vi "Generate AC Measurement Waveform.vi"(6 "hardware commands sync queue":T1, 7 "Voltage(volts)":dbl, 8 "error in":errorcluster, 9 "Frequency":dbl, 10 "DAQmx product name":string, 11 "DSG task in":refnum<k21>) -> (0 "error out":errorcluster, 3 "DSG task out":refnum<k21>)   [LabVIEW 2021]
uses:
  controls/Sync Commands Queue Ref.ctl
  controls/Sync Commands.ctl
  <vilib>/addons/_NISVFA/_Generation/Signal Generation/SV Signal/sv_System Timing Model.ctl
  <vilib>/DAQmx/write.llb/DAQmx Write (Analog 1D Wfm NChan NSamp).vi
  <vilib>/addons/_NISVFA/_Generation/Signal Generation/SV Sinusoid/SV Sinusoid.lvclass
  C:/Program Files/National Instruments/LabVIEW 2021/vi.lib/addons/_NISVFA/_Generation/Signal Generation/SV Signal/SV Signal.lvclass
  <vilib>/addons/_NISVFA/_Generation/Signal Generation/SV Sinusoid/Configure Sine.vi
  <vilib>/addons/_NISVFA/_Generation/Signal Generation/SV Signal/Write Sample Rate.vi
  <vilib>/addons/_NISVFA/_Generation/Signal Generation/SV Signal/Write System Timing Model.vi
  <vilib>/addons/_NISVFA/_Generation/Signal Generation/SV Signal/Write Ramp Parameters.vi
  <vilib>/DAQmx/miscellaneous.llb/DAQmx Fill In Error Info.vi
  <resource>/objmgr/daqmx.rc
  <vilib>/addons/_NISVFA/_Generation/Signal Generation/SV Signal/SV Signal.lvclass
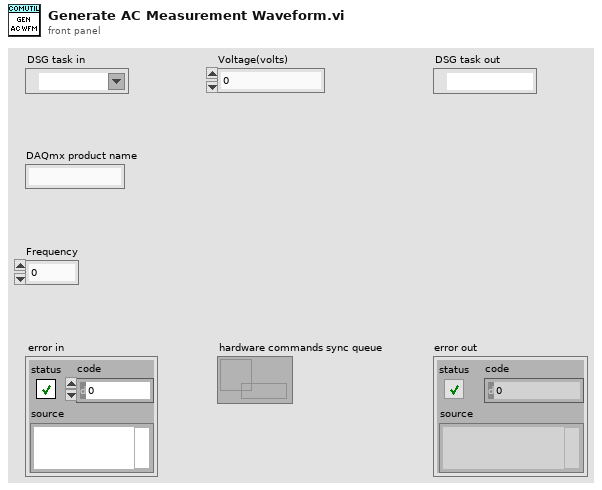
[diagram p1: front panel]
types:
  T1 = typedef "Sync Commands Queue Ref.ctl" = refnum<queue>
  T2 = typedef "Sync Commands.ctl" = enum16{"NoAction", "GenerationStarted", "AcquisitionCompleted", "GenerationErrored"}
  T3 = cluster{"profile":enum16{"Linear", "Half cosine"}, "durations [s]":cluster{"ramp-up":dbl, "transition":dbl, "ramp-down":dbl}}
  T4 = typedef "SV Signal.lvclass/sv_System Timing Model.ctl" = i64
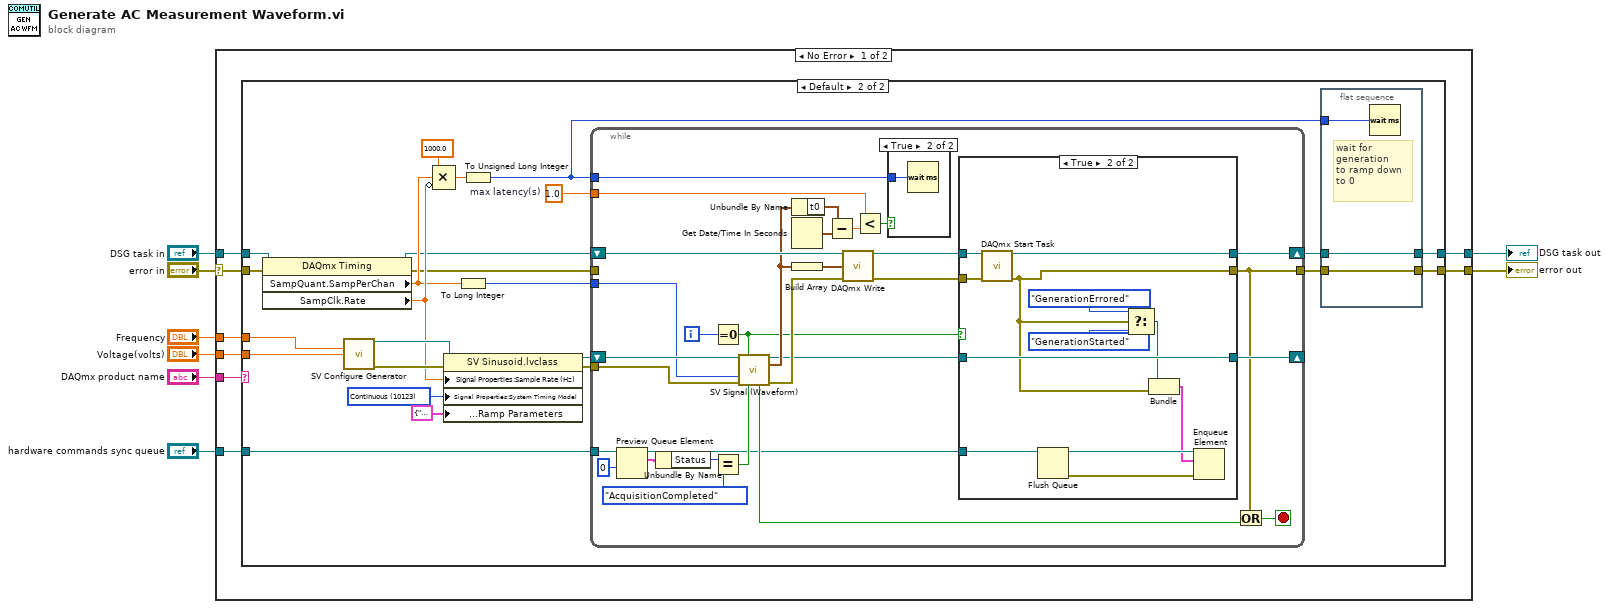
[diagram p0: block diagram]
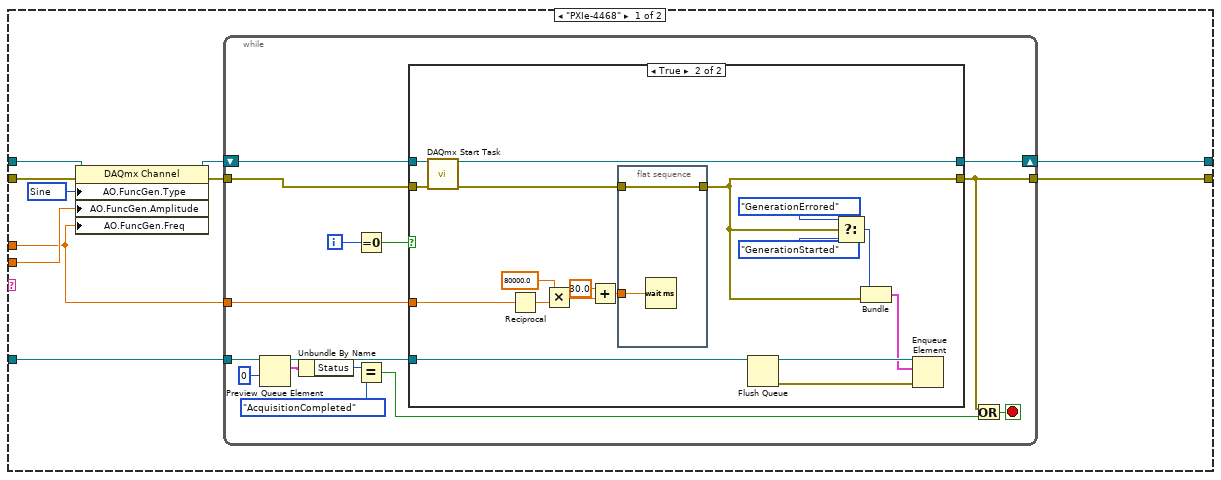
[diagram p2: hidden frame]
diagram:
  n1 = case shown="No Error" "error in" {
    selector: "error in" -> [w16 w138]
    tunnel: [w15 w137] -> w7
    tunnel: [w14 w138] -> w6
    tunnel: "DSG task in" -> [w11 w137]
    tunnel: "hardware commands sync queue" -> [w13 _]
    tunnel: "DAQmx product name" -> [w10 _]
    tunnel: "Frequency" -> [w9 _]
    tunnel: "Voltage(volts)" -> [w12 _]
    frame No Error {
      n2 = case shown="Default" w10 {
        tunnel: w16 -> [w20 w87]
        tunnel: w11 -> [w22 w83]
        tunnel: [w25 w71] -> w15
        tunnel: [w24 w70] -> w14
        tunnel: w13 -> [w26 w68]
        tunnel: w9 -> [w17 w66]
        tunnel: w12 -> [w18 w65]
        frame "PXIe-4468" {
          w19 = 14751 items=["Sine"=14751, "Triangle"=14752, "Square"=14753, "Sawtooth"=14754] ("AO.FuncGen.Type")
          n3 = property class="DAQmx Channel"(reference=w22, error in=w20, "AO.FuncGen.Type"=w19, "AO.FuncGen.Amplitude"=w18, "AO.FuncGen.Freq"=w17) -> (reference out=w23:refnum<k21>, error out=w21:errorcluster)
          n4 = while {
            tunnel: w21 -> [w40]
            shift-right: [w34] -> w25
            shift-left: w23 -> [w39]
            tunnel: [w27] -> w24
            tunnel: w26 -> [w31]
            tunnel: w17 -> [w28]
            i -> [w41]
            stop <- w38 stop-if-true
            n5 = Preview Queue Element(queue=w31, timeout in ms (-1)=0) -> (queue out=w35:T1, element=w33:cluster{"Status":T2, "Error":errorcluster})  [unwired: 1 in, 2 out]
            n6 = Unbundle By Name(w33) -> ("Status"=w32:T2)
            n7 = Equal To 0?(x=w41) -> (x = 0?=w30:bool)
            n8 = Equal?(x=w32, y=Sync_Commands."AcquisitionCompleted") -> (x = y?=w29:bool)
            n9 = case shown="True" w30 {
              tunnel: w35 -> [_ w61]
              tunnel: w39 -> [w43 w59]
              tunnel: [w43 w45] -> w34
              tunnel: w40 -> [w42 w58]
              tunnel: [w42 w47] -> w27
              tunnel: w28 -> [_ w44]
              frame False {
              }
              frame True {
                n10 = call <vilib>:"DAQmx Start Task.vi"("task/channels in"=w59, "error in"=w58) -> ("task out"=w45:refnum<k21>, "error out"=w48:errorcluster)  [unwired: 12 in]
                n11 = Reciprocal(x=w44) -> (1/x=w49:dbl)
                n12 = Multiply(x=80000.0, y=w49) -> (x*y=w51:dbl)
                n13 = Add(x=30.0, y=w51) -> (x+y=w46:dbl)
                n14 = flat-sequence {
                  tunnel: w48 -> [w63]
                  tunnel: [w63] -> w47
                  tunnel: w46 -> [w62]
                  frame #0 {
                    n15 = Wait (ms)(milliseconds to wait=w62) -> ()  [unwired: 1 out]
                  }
                }
                n16 = Flush Queue(queue=w61) -> (queue out=w60:T1, error out=w57:errorcluster)  [unwired: 1 in, 1 out]
                n17 = Select(t=Sync_Commands."GenerationErrored" ("element"), s=w47, f=Sync_Commands."GenerationStarted" ("element")) -> (s? t:f=w54:T2)
                n18 = Bundle("element"=w54, "error out"=w47) -> (w53:cluster{"element":T2, "error out":errorcluster})  [unwired: 1 in]
                n19 = Enqueue Element(queue=w60, element=w53, error in (no error)=w57) -> ()  [unwired: 1 in, 3 out]
              }
            }
            n20 = Or(x=w27, y=w29) -> (x .or. y?=w38:bool)
          }
        }
        frame Default {
          w76 = 1.0  # max latency(s)
          w84 = T4 10123 items=["Finite"=10178, "-"=-1, "Continuous"=10123, "-"=-2, "Settled"=110123, "Averaged"=210123, "Discrete Sweep"=310123, "Continuous Sweep"=410123] ("System Timing Model")
          n21 = property class="DAQmx Timing"(reference=w83, error in=w87) -> (reference out=w77:refnum<k21>, error out=w64:errorcluster, "SampQuant.SampPerChan"=w79:dbl, "SampClk.Rate"=w82:dbl)
          n22 = call-poly <vilib>:"SV Configure Generator.vi"("frequency (Hz)"=w66, "amplitude"=w65) -> ("signal configuration"=w85:refnum<class "SV Sinusoid.lvclass">, "error out"=w86:errorcluster)  [unwired: 12 in]
          n23 = Compound Arithmetic op=MULTIPLY(1000.0 ("value"), w79, invert w82) -> (w75:dbl)
          n24 = property class="SV Sinusoid.lvclass"(reference=w85, error in=w86, "Signal Properties:Sample Rate (Hz)"=w82, "Signal Properties:System Timing Model"=w84, "Signal Properties:Ramps:Ramp Parameters"=T3 {"profile"=enum."Linear", "durations [s]"={"ramp-up"=0.0, "transition"=0.0, "ramp-down"=0.01}} ("Ramp Parameters:All Elements")) -> (reference out=w81:refnum<class "SV Sinusoid.lvclass">, error out=w80:errorcluster)
          n25 = To Long Integer(number=w79) -> (32bit integer=w78:i32)
          n26 = To Unsigned Long Integer(number=w75) -> (unsigned 32bit integer=w69:u32)
          n27 = while {
            shift-right: [w94] -> _
            shift-left: w81 -> [w120]
            tunnel: w80 -> [w117]
            tunnel: w78 -> [w118]
            shift-right: [w97] -> w72
            shift-left: w77 -> [w116]
            tunnel: [w91] -> w73
            tunnel: w76 -> [w107]
            tunnel: w69 -> [w105]
            tunnel: w68 -> [w104]
            tunnel: w64 -> [_]
            i -> [w119]
            stop <- w112 stop-if-true
            n28 = Preview Queue Element(queue=w104, timeout in ms (-1)=0) -> (queue out=w100:T1, element=w93:cluster{"Status":T2, "Error":errorcluster})  [unwired: 1 in, 2 out]
            n29 = Unbundle By Name(w93) -> ("Status"=w92:T2)
            n30 = Equal To 0?(x=w119) -> (x = 0?=w99:bool)
            n31 = Equal?(x=w92, y=Sync_Commands."AcquisitionCompleted") -> (x = y?=w101:bool)
            n32 = call-dynamic "SV Signal (Waveform).vi"("signal configuration"=w120, "reset"=w99, "samples"=w118, "error in (no error)"=w117, "stop"=w101) -> ("signal configuration"=w95:refnum<class "SV Sinusoid.lvclass">, "output waveform"=w111:waveform(dbl), "done"=w113:bool, "error out"=w114:errorcluster)  [unwired: 5 in, 2 out]
            n33 = Unbundle By Name(w111) -> ("t0"=w110:timestamp)
            n34 = Get Date/Time In Seconds() -> (seconds since 1Jan1904=w109:timestamp)
            n35 = Build Array(w111) -> (w115:waveform(dbl)[])
            n36 = Subtract(x=w110, y=w109) -> (x-y=w108:dbl)
            n37 = call-poly <vilib>:"DAQmx Write.vi"("task/channels in"=w116, "data"=w115, "error in"=w114) -> ("task out"=w98:refnum<k21>, "error out"=w96:errorcluster)  [unwired: 10 in, 1 out]
            n38 = Less?(x=w107, y=w108) -> (x < y?=w106:bool)
            n39 = case shown="True" w106 {
              tunnel: w105 -> [_ w136]
              frame False {
              }
              frame True {
                n40 = Wait (ms)(milliseconds to wait=w136) -> ()  [unwired: 1 out]
              }
            }
            n41 = case shown="True" w99 {
              tunnel: w100 -> [_ w135]
              tunnel: w98 -> [w123 w133]
              tunnel: [w123 w132] -> w97
              tunnel: w96 -> [w122 w131]
              tunnel: [w122 w125] -> w91
              tunnel: w95 -> [w121 w127]
              tunnel: [w121 w127] -> w94
              frame False {
              }
              frame True {
                n42 = call <vilib>:"DAQmx Start Task.vi"("task/channels in"=w133, "error in"=w131) -> ("task out"=w132:refnum<k21>, "error out"=w125:errorcluster)  [unwired: 12 in]
                n43 = Flush Queue(queue=w135) -> (queue out=w134:T1, error out=w130:errorcluster)  [unwired: 1 in, 1 out]
                n44 = Select(t=Sync_Commands."GenerationErrored" ("element"), s=w125, f=Sync_Commands."GenerationStarted" ("element")) -> (s? t:f=w126:T2)
                n45 = Bundle("element"=w126, "error out"=w125) -> (w124:cluster{"element":T2, "error out":errorcluster})  [unwired: 1 in]
                n46 = Enqueue Element(queue=w134, element=w124, error in (no error)=w130) -> ()  [unwired: 1 in, 3 out]
              }
            }
            n47 = Or(x=w91, y=w113) -> (x .or. y?=w112:bool)
          }
          n48 = flat-sequence {
            tunnel: w73 -> [w89]
            tunnel: w72 -> [w90]
            tunnel: [w90] -> w71
            tunnel: [w89] -> w70
            tunnel: w69 -> [w88]
            frame #0 {
              # "wait for\ngeneration\nto ramp down\nto 0"
              n49 = Wait (ms)(milliseconds to wait=w88) -> ()  [unwired: 1 out]
            }
          }
        }
      }
    }
    frame Error {
    }
  }
  "DSG task out" <- w7
  "error out" <- w6
